vi "Process_One_Second.vi"(6 "Queues":T12, 7 "One Seconds in":T10[](array[typedef]) {"Ch1 High" format="%0.0f"}, 8 "Status/Errors in":refnum<vi>, 9 "Process data parameters in":T1={"Stop loop"={"Settings changed?"=FALSE, "Stop?"=refnum}, "Button refs"={"Stop program"=refnum, "Save settings"=refnum, "DAQ mode"=refnum, "Reset settings"=refnum, "Apply settings"=refnum, "Reset MAS"=refnum, "Reset SLV"=refnum, "Local DBase?"=refnum, "Last value DBase"=FALSE, "Database"=refnum, "Calibration"=refnum, "Save settings 2"=refnum}, "Process messages"={"Process message mode"=enum."Error", "Slave data?"=FALSE, "Length get settings message"=0, "Delta time"=0.0, "Data_Filter"={"Filter_Data"=FALSE, "Use_Thresh"=FALSE, "Reduce data?"=FALSE}, "Time_difference_stack"=[], "Starting sec"=0, "Ending sec"=0, "Ending sec 2"=0, "MAS_Page_Thresh"=refnum, "SLV_Page_Thresh"=refnum, "Database"=refnum}, "Settings state"={"MAS locked?"=refnum, "SLV locked?"=refnum}, "Mode"={"Mode"=enum."Dialog", "Expert?"=FALSE, "Dialog?"=FALSE}, "Alignment parameters"=refnum, "Timer parameters"=refnum, "Files"={"Path config file"=path "", "Path def. ini file"=path "", "Path ini file 1"=path "", "Path ini file 2"=path "", "Path RBF file"=path ""}, "Time difference"=refnum, "Alignment"={"GEN_Page_Calibrate"=refnum, "MAS_Page_Gain"=refnum, "MAS_Page_Offset"=refnum, "SLV_Page_Gain"=refnum, "SLV_Page_Offset"=refnum, "MAS_Page_Common"=refnum, "SLV_Page_Common"=refnum}, "Page Statistics"=refnum}, 11 "Device in":refnum<vi>) -> (0 "Status/Errors out":refnum<vi>, 3 "Device out":refnum<vi>, 5 "One Seconds out":T10[](array[typedef]) {"Ch1 High" format="%0.0f"})   [LabVIEW 2010]
uses:
  Controls/Queues.ctl
  Controls/One_Second.ctl
  Controls/GPS_Timestamp.ctl
  Controls/Process_Data_Parameters.ctl
  Controls/Stop_Loop.ctl
  Controls/Button_Refs.ctl
  Controls/Process_Messages.ctl
  Controls/Process_Message_Mode.ctl
  Controls/Settings_State.ctl
  Controls/Mode.ctl
  Controls/Files.ctl
  Controls/Page_Calibration.ctl
  Controls/Device_Elements.ctl
  Controls/Get_Set_Device_Options.ctl
  Controls/Get_Set_Timer_Options.ctl
  Controls/Add_Subtract.ctl
  Controls/Master.ctl
  Controls/Configuration_File_Parameters.ctl
  Controls/Timer_Elements.ctl
  Controls/Configuration_File_Elements.ctl
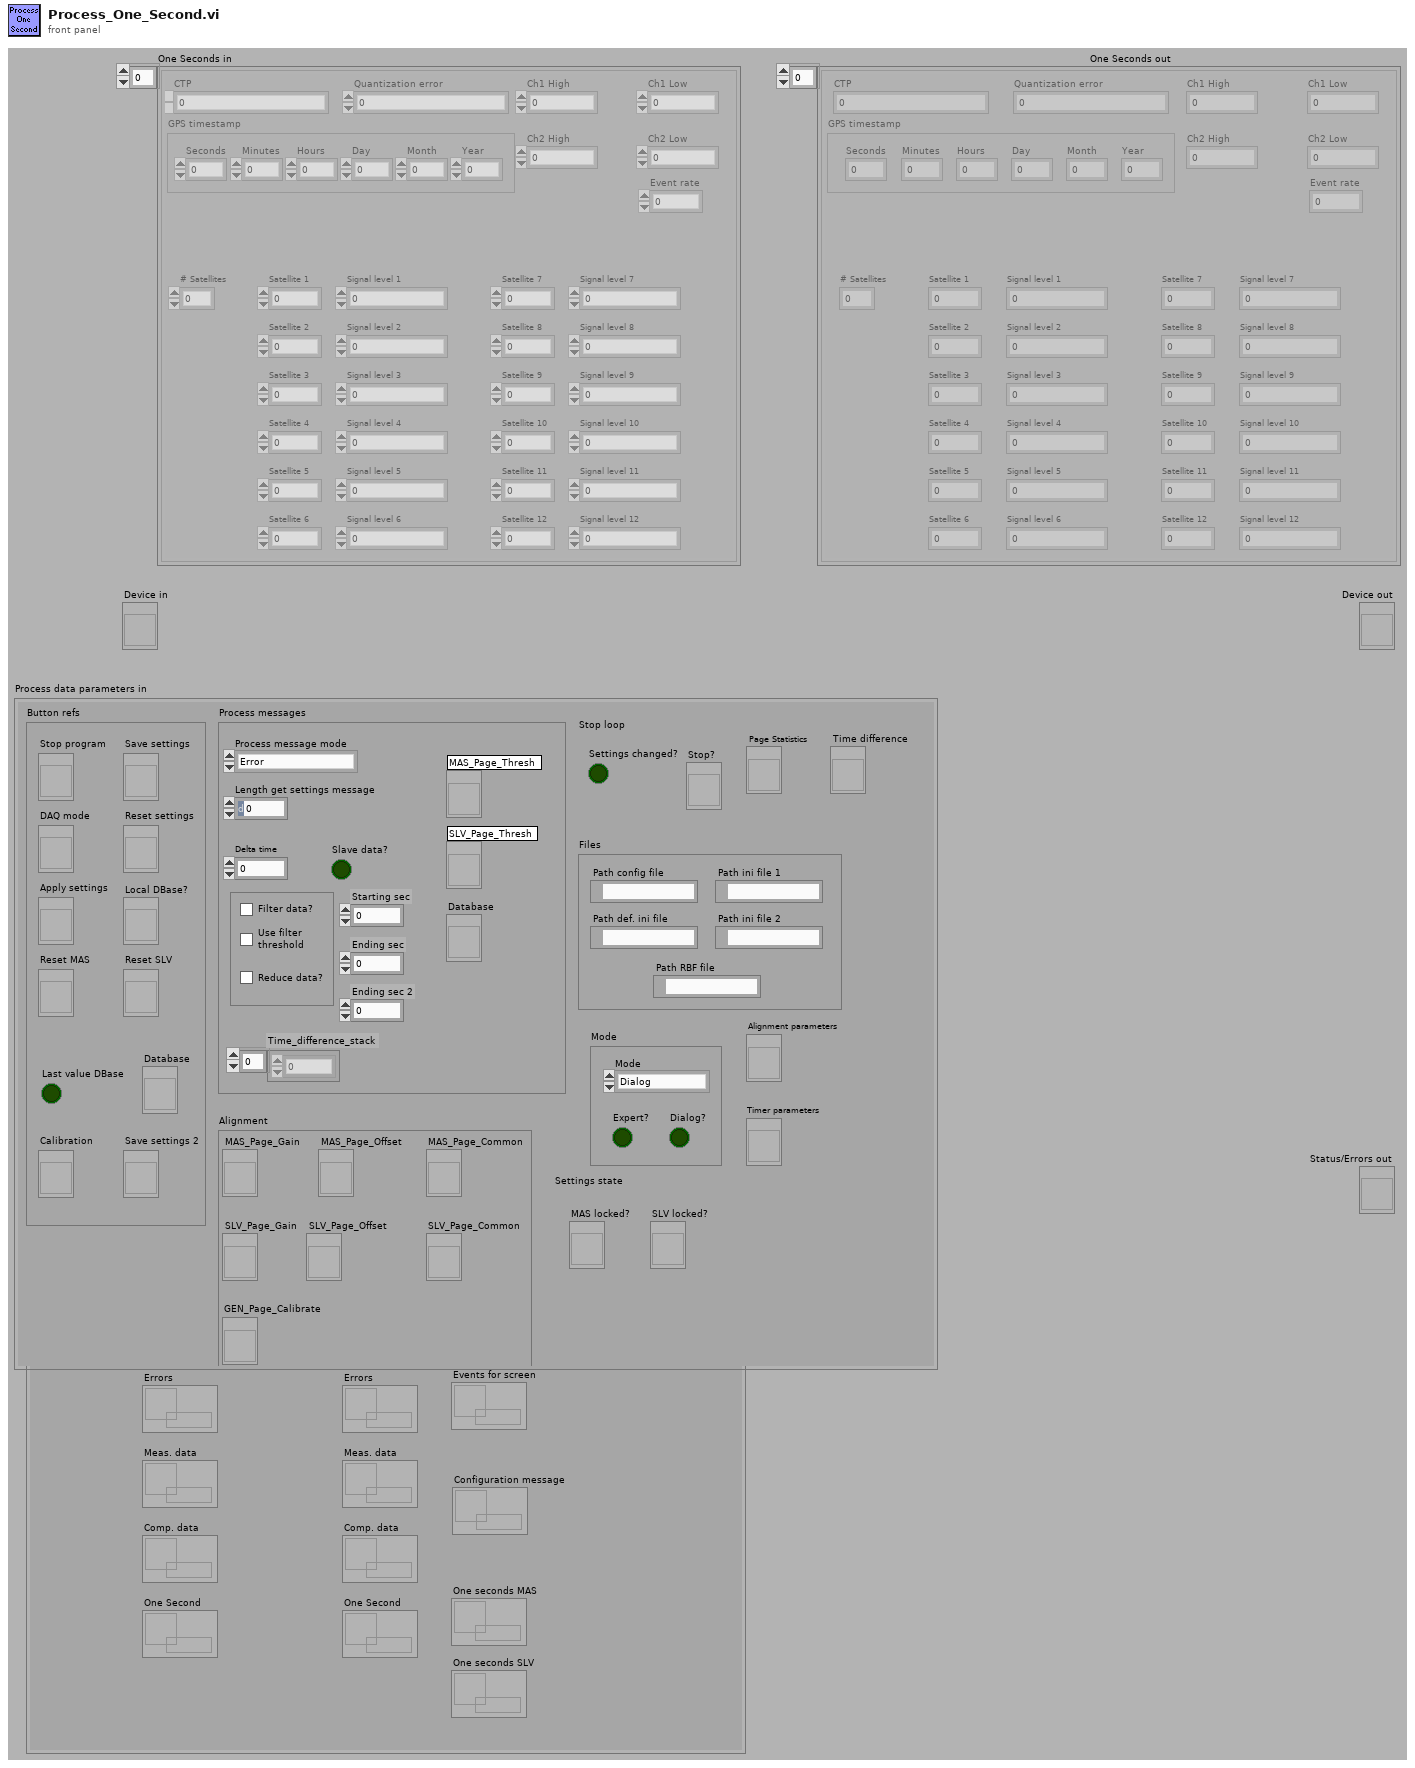
[diagram p1: front panel]
types:
  T1 = typedef "Process_Data_Parameters.ctl" = cluster{"Stop loop":T2, "Button refs":T3, "Process messages":T4, "Settings state":T6, "Mode":T7, "Alignment parameters":refnum<vi>, "Timer parameters":refnum<vi>, "Files":T8, "Time difference":refnum<vi>, "Alignment":T9, "Page Statistics":refnum<vi>}
  T2 = typedef "Stop_Loop.ctl" = cluster{"Settings changed?":bool, "Stop?":refnum<vi>}
  T3 = typedef "Button_Refs.ctl" = cluster{"Stop program":refnum<vi>, "Save settings":refnum<vi>, "DAQ mode":refnum<vi>, "Reset settings":refnum<vi>, "Apply settings":refnum<vi>, "Reset MAS":refnum<vi>, "Reset SLV":refnum<vi>, "Local DBase?":refnum<vi>, "Last value DBase":bool, "Database":refnum<vi>, "Calibration":refnum<vi>, "Save settings 2":refnum<vi>}
  T4 = typedef "Process_Messages.ctl" = cluster{"Process message mode":T5, "Slave data?":bool, "Length get settings message":i32, "Delta time":dbl, "Data_Filter":cluster{"Filter_Data":bool, "Use_Thresh":bool, "Reduce data?":bool}, "Time_difference_stack":u64[], "Starting sec":u64, "Ending sec":u64, "Ending sec 2":u64, "MAS_Page_Thresh":refnum<vi>, "SLV_Page_Thresh":refnum<vi>, "Database":refnum<vi>}
  T5 = typedef "Process_Message_Mode.ctl" = enum16{"Error", "Measurement data", "Comparator data", "One Second"}
  T6 = typedef "Settings_State.ctl" = cluster{"MAS locked?":refnum<vi>, "SLV locked?":refnum<vi>}
  T7 = typedef "Mode.ctl" = cluster{"Mode":enum8{"Stop", "Dialog", "Hisparc II", "Hisparc II DAQ", "Alignment"}, "Expert?":bool, "Dialog?":bool}
  T8 = typedef "Files.ctl" = cluster{"Path config file":path, "Path def. ini file":path, "Path ini file 1":path, "Path ini file 2":path, "Path RBF file":path}
  T9 = typedef "Page_Calibration.ctl" = cluster{"GEN_Page_Calibrate":refnum<vi>, "MAS_Page_Gain":refnum<vi>, "MAS_Page_Offset":refnum<vi>, "SLV_Page_Gain":refnum<vi>, "SLV_Page_Offset":refnum<vi>, "MAS_Page_Common":refnum<vi>, "SLV_Page_Common":refnum<vi>}
  T10 = typedef "One_Second.ctl" = cluster{"GPS timestamp":T11, "CTP":u32, "Quantization error":u32, "Ch1 High":u16, "Ch1 Low":u16, "Ch2 High":u16, "Ch2 Low":u16, "Event rate":u16, "# Satellites":u8, "Satellite 1":u8, "Satellite 2":u8, "Satellite 3":u8, "Satellite 4":u8, "Satellite 5":u8, "Satellite 6":u8, "Signal level 1":sgl, "Signal level 2":sgl, "Signal level 3":sgl, "Signal level 4":sgl, "Signal level 5":sgl, "Signal level 6":sgl, "Satellite 7":u8, "Satellite 8":u8, "Satellite 9":u8, "Satellite 10":u8, "Satellite 11":u8, "Satellite 12":u8, "Signal level 7":sgl, "Signal level 8":sgl, "Signal level 9":sgl, "Signal level 10":sgl, "Signal level 11":sgl, "Signal level 12":sgl}
  T11 = typedef "GPS_Timestamp.ctl" = cluster{"Seconds":u8, "Minutes":u8, "Hours":u8, "Day":u8, "Month":u8, "Year":u16}
  T12 = typedef "Queues.ctl" = cluster{"MAS":cluster{"Bytes":refnum<queue>, "Settings":refnum<queue>, "Errors":refnum<queue>, "Meas. data":refnum<queue>, "One Second":refnum<queue>, "Comp. data":refnum<queue>}, "SLV":cluster{"Bytes":refnum<queue>, "Settings":refnum<queue>, "Errors":refnum<queue>, "Meas. data":refnum<queue>, "One Second":refnum<queue>, "Comp. data":refnum<queue>}, "Events to store":refnum<queue>, "Events for screen":refnum<queue>, "One seconds MAS":refnum<queue>, "One seconds SLV":refnum<queue>, "Configuration message":refnum<queue>, "Comparator to store":refnum<queue>}
  T13 = typedef "Get_Set_Device_Options.ctl" = enum16{"Get", "Get cluster", "Set"}
  T14 = typedef "Device_Elements.ctl" = enum16{"Default", "Master?", "Connected?", "Status", "Disconnect?", "Handle", "Version number"}
  T15 = typedef "Master.ctl" = enum16{"Master", "Slave", "General"}
  T16 = typedef "Get_Set_Timer_Options.ctl" = enum16{"Get", "Get cluster", "Set", "Set to current time"}
  T17 = typedef "Timer_Parameters.ctl" = cluster{"current time (ms)":u32, "time (ms) screen updated":u32, "time (ms) controls locked":u32, "time (ms) last device check":u32, "time (ms) last data MAS":u32, "time (ms) last data SLV":u32, "time (ms) bad status MAS":u32, "time (ms) bad status SLV":u32, "time (ms) clock error updated":u32, "time delay screen update (ms)":u32, "time delay controls (ms)":u32, "time delay device check (ms)":u32, "time until MAS status bad (ms)":u32, "time until SLV status bad (ms)":u32, "time until MAS connection bad (ms)":u32, "time until SLV connection bad (ms)":u32, "time delay clock error update (ms)":u32}
  T18 = cluster{"[0]":u8, "[1]":u8, "[2]":u8, "[3]":u8, "[4]":u8, "[5]":u8, "[6]":u8}
  T19 = cluster{"[0]":u8, "[1]":u8, "[2]":u8, "[3]":u8, "[4]":u8, "[5]":u8, "[6]":u8, "[7]":u8}
  T20 = cluster{"second":i32, "minute":i32, "hour":i32, "day of month":i32, "month":i32, "year":i32, "day of week":i32, "day of year":i32, "is DST":i32}
  T21 = typedef "Add_Subtract.ctl" = enum16{"Add", "Subtract"}
  T22 = typedef "Configuration_File_Parameters.ctl" = cluster{"Mode":T7, "Hardware":enum8{"None", "HiSPARC I", "HiSPARC II", "HiSPARC III"}, "Time difference":string}
  T23 = typedef "Timer_Elements.ctl" = enum16{"Default", "Current time", "Time screen updated", "Time controls locked", "Time last device check", "Time last data MAS", "Time last data SLV", "Time bad status MAS", "Time bad status SLV", "Time clock error updated", "Time delay screen update", "Time delay controls", "Time delay device check", "Time until MAS status bad", "Time until SLV status bad", "Time until MAS connection bad", "Time until SLV connection bad", "Time delay clock error update"}
  T24 = typedef "Configuration_File_Elements.ctl" = enum16{"None", "All", "Mode", "Hardware", "Time difference"}
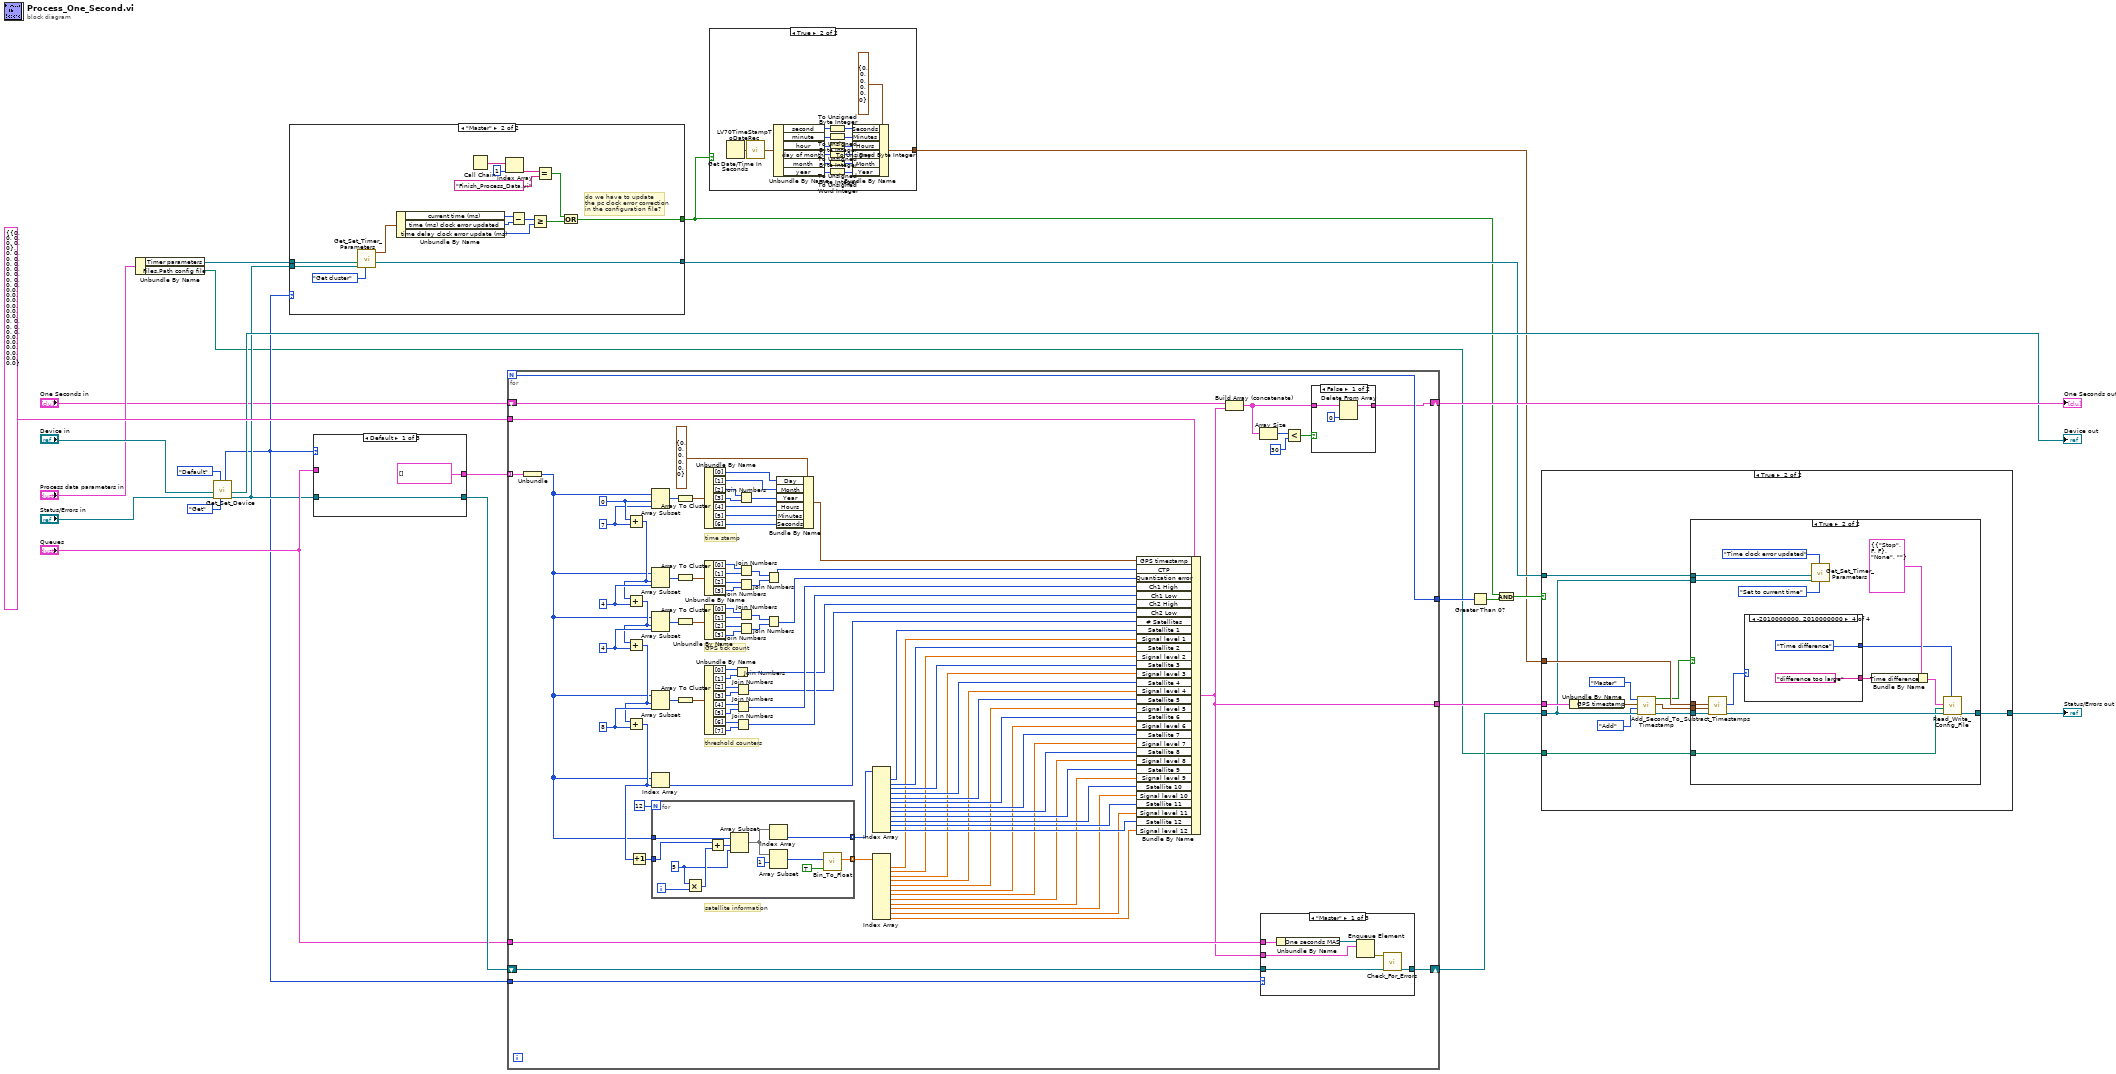
[diagram p0: block diagram]
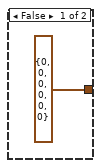
[diagram p2: hidden frame]
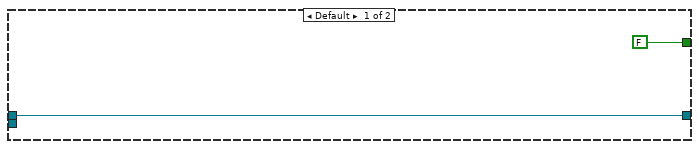
[diagram p3: hidden frame]
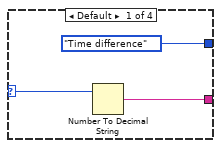
[diagram p6: hidden frame]
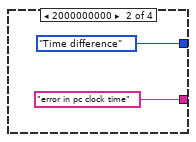
[diagram p7: hidden frame]
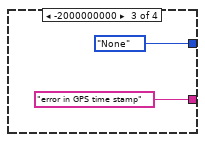
[diagram p8: hidden frame]
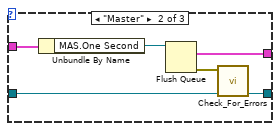
[diagram p9: hidden frame]
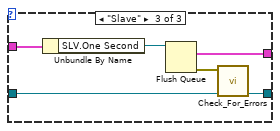
[diagram p10: hidden frame]
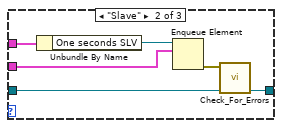
[diagram p12: hidden frame]
diagram:
  n1 = Unbundle By Name("Process data parameters in") -> ("Timer parameters"=w5:refnum<vi>, "Files.Path config file"=w1:path)
  n2 = call "Get_Set_Device.vi"("Get/Set"=Get_Set_Device_Options."Get", "Element"=Device_Elements."Default", "Status/Errors in"="Status/Errors in", "Device in"="Device in") -> ("Status/Errors out"=w8:refnum<vi>, "Device out"=→"Device out":refnum<vi>, "Master?"=w7:T15)  [unwired: 1 in, 4 out]
  n3 = case shown="\"Master\"" w7 {
    tunnel: w5 -> [w26 w33]
    tunnel: [w26 w38] -> w11
    tunnel: [FALSE w35] -> w4
    tunnel: w8 -> [_ w34]
    frame Default {
    }
    frame "Master" {
      # "do we have to update\nthe pc clock error correction\nin the configuration file?"
      n4 = call "Get_Set_Timer_Parameters.vi"("Get/Set"=Get_Set_Timer_Options."Get cluster", "Status/Errors in"=w34, "Timer parameters in"=w33) -> ("Timer parameters out"=w38:refnum<vi>, "Timer cluster"=w37:T17)  [unwired: 2 in, 5 out]
      n5 = Unbundle By Name(w37) -> ("current time (ms)"=w29:u32, "time (ms) clock error updated"=w30:u32, "time delay clock error update (ms)"=w31:u32)
      n6 = Call Chain() -> (call chain=w43:string[])
      n7 = Index Array(array=w43, index=1) -> (element=w41:string)
      n8 = Subtract(x=w29, y=w30) -> (x-y=w32:u32)
      n9 = Greater Or Equal?(x=w32, y=w31) -> (x >= y?=w28:bool)
      n10 = Equal?(x=w41, y="Finish_Process_Data.vi") -> (x = y?=w36:bool)
      n11 = Or(x=w36, y=w28) -> (x .or. y?=w35:bool)
    }
  }
  n12 = case shown="Default" w7 {
    tunnel: "Queues" -> [_ w51 w57]
    tunnel: [cluster{u8[]}[] [] ("remaining elements") w50 w56] -> w22
    tunnel: w8 -> [w44 w47 w53]
    tunnel: [w44 w46 w52] -> w20
    frame Default {
    }
    frame "Master" {
      n13 = Unbundle By Name(w51) -> ("MAS.One Second"=w49:refnum<queue>)
      n14 = Flush Queue(queue=w49) -> (remaining elements=w50:cluster{u8[]}[], error out=w48:errorcluster)  [unwired: 1 in, 1 out]
      n15 = call "Check_For_Errors.vi"("Status/Errors in"=w47, "error in"=w48) -> ("Status/Errors out"=w46:refnum<vi>)  [unwired: 9 out]
    }
    frame "Slave" {
      n16 = Unbundle By Name(w57) -> ("SLV.One Second"=w55:refnum<queue>)
      n17 = Flush Queue(queue=w55) -> (remaining elements=w56:cluster{u8[]}[], error out=w54:errorcluster)  [unwired: 1 in, 1 out]
      n18 = call "Check_For_Errors.vi"("Status/Errors in"=w53, "error in"=w54) -> ("Status/Errors out"=w52:refnum<vi>)  [unwired: 9 out]
    }
  }
  n19 = for {
    N -> [w72]
    tunnel: w22 -> [w111] mode=indexing
    shift-right: [w66] -> w23
    shift-left: "One Seconds in" -> [w68]
    tunnel: T10 {"GPS timestamp"={"Seconds"=0, "Minutes"=0, "Hours"=0, "Day"=0, "Month"=0, "Year"=0}, "CTP"=0, "Quantization error"=0, "Ch1 High"=0, "Ch1 Low"=0, "Ch2 High"=0, "Ch2 Low"=0, "Event rate"=0, "# Satellites"=0, "Satellite 1"=0, "Satellite 2"=0, "Satellite 3"=0, "Satellite 4"=0, "Satellite 5"=0, "Satellite 6"=0, "Signal level 1"=0.0, "Signal level 2"=0.0, "Signal level 3"=0.0, "Signal level 4"=0.0, "Signal level 5"=0.0, "Signal level 6"=0.0, "Satellite 7"=0, "Satellite 8"=0, "Satellite 9"=0, "Satellite 10"=0, "Satellite 11"=0, "Satellite 12"=0, "Signal level 7"=0.0, "Signal level 8"=0.0, "Signal level 9"=0.0, "Signal level 10"=0.0, "Signal level 11"=0.0, "Signal level 12"=0.0} ("GPS Tick Count Message") -> [w110]
    tunnel: w7 -> [w75]
    tunnel: "Queues" -> [w74]
    tunnel: [w69] -> w16
    shift-right: [w73] -> w13
    shift-left: w20 -> [w76]
    tunnel: [w72] -> w10
    w109 = 8 ("y")
    w115 = 4 ("y")
    w116 = 4 ("y")
    w117 = 7 ("y")
    w118 = 0
    # "satellite information"
    # "time stamp"
    # "GPS tick count"
    # "threshold counters"
    n20 = Unbundle(w111) -> (w103:u8[])
    n21 = Add(x=w118, y=w117) -> (x+y=w114:i32)
    n22 = Add(x=w114, y=w116) -> (x+y=w113:i32)
    n23 = Add(x=w113, y=w115) -> (x+y=w108:i32)
    n24 = Add(x=w108, y=w109) -> (x+y=w107:i32)
    n25 = Increment(x=w107) -> (x+1=w106:i32)
    n26 = Array Subset(array=w103, index=w118, length=w117) -> (w154:u8[])
    n27 = Array Subset(array=w103, index=w114, length=w116) -> (w129:u8[])
    n28 = Array Subset(array=w103, index=w113, length=w115) -> (w130:u8[])
    n29 = Array Subset(array=w103, index=w108, length=w109) -> (w128:u8[])
    n30 = Index Array(array=w103, index=w107) -> (element=w105:u8)
    n31 = for {
      N: 12 -> [_]
      tunnel: w106 -> [w176]
      tunnel: w103 -> [w179]
      tunnel: [w174] -> w102 mode=indexing
      tunnel: [w173] -> w89 mode=indexing
      i -> [w178]
      w172 = 5 ("x")
      n32 = Multiply(x=w172, y=w178) -> (x*y=w175:i32)
      n33 = Add(x=w176, y=w175) -> (x+y=w177:i32)
      n34 = Array Subset(array=w179, index=w177, length=w172) -> (w183:u8[])
      n35 = Index Array(array=w183) -> (element=w174:u8)  [unwired: 1 in]
      n36 = Array Subset(array=w183, index=1) -> (w181:u8[])  [unwired: 1 in]
      n37 = call "Bin_To_Float.vi"("32 Bit?"=TRUE, "Binary float"=w181) -> ("Single-Precision Float"=w173:sgl)  [unwired: 9 out]
    }
    n38 = Array To Cluster(array=w154) -> (cluster=w138:T18)
    n39 = Array To Cluster(array=w129) -> (cluster=w131:cluster{"[0]":u8, "[1]":u8, "[2]":u8, "[3]":u8})
    n40 = Array To Cluster(array=w130) -> (cluster=w143:cluster{"[0]":u8, "[1]":u8, "[2]":u8, "[3]":u8})
    n41 = Array To Cluster(array=w128) -> (cluster=w123:T19)
    n42 = Unbundle By Name(w138) -> ("[0]"=w150:u8, "[1]"=w149:u8, "[2]"=w152:u8, "[3]"=w151:u8, "[4]"=w147:u8, "[5]"=w146:u8, "[6]"=w112:u8)
    n43 = Unbundle By Name(w131) -> ("[0]"=w134:u8, "[1]"=w136:u8, "[2]"=w135:u8, "[3]"=w137:u8)
    n44 = Unbundle By Name(w143) -> ("[0]"=w142:u8, "[1]"=w140:u8, "[2]"=w141:u8, "[3]"=w139:u8)
    n45 = Unbundle By Name(w123) -> ("[0]"=w127:u8, "[1]"=w125:u8, "[2]"=w126:u8, "[3]"=w124:u8, "[4]"=w122:u8, "[5]"=w121:u8, "[6]"=w120:u8, "[7]"=w119:u8)
    n46 = Join Numbers(hi=w127, lo=w125) -> ((hi.lo)=w59:u16)
    n47 = Join Numbers(hi=w126, lo=w124) -> ((hi.lo)=w58:u16)
    n48 = Join Numbers(hi=w122, lo=w121) -> ((hi.lo)=w61:u16)
    n49 = Join Numbers(hi=w120, lo=w119) -> ((hi.lo)=w60:u16)
    n50 = Join Numbers(hi=w152, lo=w151) -> ((hi.lo)=w148:u16)
    n51 = Join Numbers(hi=w134, lo=w136) -> ((hi.lo)=w132:u16)
    n52 = Join Numbers(hi=w135, lo=w137) -> ((hi.lo)=w133:u16)
    n53 = Join Numbers(hi=w142, lo=w140) -> ((hi.lo)=w145:u16)
    n54 = Join Numbers(hi=w141, lo=w139) -> ((hi.lo)=w144:u16)
    n55 = Join Numbers(hi=w132, lo=w133) -> ((hi.lo)=w63:u32)
    n56 = Join Numbers(hi=w145, lo=w144) -> ((hi.lo)=w62:u32)
    n57 = Bundle By Name(cluster=T11 {"Seconds"=0, "Minutes"=0, "Hours"=0, "Day"=0, "Month"=0, "Year"=0} ("GPS timestamp in"), "Day"=w150, "Month"=w149, "Year"=w148, "Hours"=w147, "Minutes"=w146, "Seconds"=w112) -> (w64:T11)
    n58 = Index Array(array=w102) -> (element #1=w90:u8, element #2=w91:u8, element #3=w92:u8, element #4=w93:u8, element #5=w94:u8, element #6=w95:u8, element #7=w96:u8, element #8=w97:u8, element #9=w98:u8, element #10=w99:u8, element #11=w100:u8, element #12=w101:u8)  [unwired: 12 in]
    n59 = Index Array(array=w89) -> (element #1=w77:sgl, element #2=w78:sgl, element #3=w79:sgl, element #4=w80:sgl, element #5=w81:sgl, element #6=w82:sgl, element #7=w83:sgl, element #8=w84:sgl, element #9=w85:sgl, element #10=w86:sgl, element #11=w87:sgl, element #12=w88:sgl)  [unwired: 12 in]
    n60 = Bundle By Name(cluster=w110, "GPS timestamp"=w64, "CTP"=w63, "Quantization error"=w62, "Ch1 High"=w61, "Ch1 Low"=w60, "Ch2 High"=w59, "Ch2 Low"=w58, "# Satellites"=w105, "Satellite 1"=w90, "Signal level 1"=w77, "Satellite 2"=w91, "Signal level 2"=w78, "Satellite 3"=w92, "Signal level 3"=w79, "Satellite 4"=w93, "Signal level 4"=w80, "Satellite 5"=w94, "Signal level 5"=w81, "Satellite 6"=w95, "Signal level 6"=w82, "Satellite 7"=w96, "Signal level 7"=w83, "Satellite 8"=w97, "Signal level 8"=w84, "Satellite 9"=w98, "Signal level 9"=w85, "Satellite 10"=w99, "Signal level 10"=w86, "Satellite 11"=w100, "Signal level 11"=w87, "Satellite 12"=w101, "Signal level 12"=w88) -> (w69:T10)
    n61 = Build Array (concatenate)(w68, w69) -> (w65:T10[])
    n62 = Array Size(array=w65) -> (size(s)=w71:i32)
    n63 = case shown="\"Master\"" w75 {
      tunnel: w76 -> [w159 w165 w171]
      tunnel: [w164 w170 w171] -> w73
      tunnel: w74 -> [w163 w169 _]
      tunnel: w69 -> [w160 w166 _]
      frame "Master" {
        n64 = Unbundle By Name(w163) -> ("One seconds MAS"=w162:refnum<queue>)
        n65 = Enqueue Element(queue=w162, element=w160) -> (error out=w161:errorcluster)  [unwired: 1 in, 3 out]
        n66 = call "Check_For_Errors.vi"("Status/Errors in"=w159, "error in"=w161) -> ("Status/Errors out"=w164:refnum<vi>)  [unwired: 9 out]
      }
      frame "Slave" {
        n67 = Unbundle By Name(w169) -> ("One seconds SLV"=w168:refnum<queue>)
        n68 = Enqueue Element(queue=w168, element=w166) -> (error out=w167:errorcluster)  [unwired: 1 in, 3 out]
        n69 = call "Check_For_Errors.vi"("Status/Errors in"=w165, "error in"=w167) -> ("Status/Errors out"=w170:refnum<vi>)  [unwired: 9 out]
      }
      frame Default {
      }
    }
    n70 = Less?(x=w71, y=30 ("x")) -> (x < y?=w67:bool)
    n71 = case shown="False" w67 {
      tunnel: [w156 w158] -> w66
      tunnel: w65 -> [w157 w158]
      frame False {
        n72 = Delete From Array(array=w157, index=0) -> (array with subset deleted=w156:T10[])  [unwired: 1 in, 1 out]
      }
      frame True {
      }
    }
  }
  "One Seconds out" <- w23
  n73 = case shown="True" w4 {
    tunnel: [T11 {"Seconds"=0, "Minutes"=0, "Hours"=0, "Day"=0, "Month"=0, "Year"=0} ("GPS timestamp") w186] -> w3
    frame False {
    }
    frame True {
      n74 = Get Date/Time In Seconds() -> (seconds since 1Jan1904=w185:timestamp)
      n75 = call <vilib>:"LV70TimeStampToDateRec.vi"("time stamp"=w185) -> ("date time rec"=w200:T20)
      n76 = Unbundle By Name(w200) -> ("second"=w198:i32, "minute"=w197:i32, "hour"=w196:i32, "day of month"=w195:i32, "month"=w194:i32, "year"=w193:i32)
      n77 = To Unsigned Byte Integer(number=w198) -> (unsigned 8bit integer=w187:u8)
      n78 = To Unsigned Byte Integer(number=w197) -> (unsigned 8bit integer=w188:u8)
      n79 = To Unsigned Byte Integer(number=w196) -> (unsigned 8bit integer=w189:u8)
      n80 = To Unsigned Byte Integer(number=w195) -> (unsigned 8bit integer=w190:u8)
      n81 = To Unsigned Byte Integer(number=w194) -> (unsigned 8bit integer=w191:u8)
      n82 = To Unsigned Word Integer(number=w193) -> (unsigned 16bit integer=w192:u16)
      n83 = Bundle By Name(cluster=T11 {"Seconds"=0, "Minutes"=0, "Hours"=0, "Day"=0, "Month"=0, "Year"=0} ("GPS timestamp"), "Seconds"=w187, "Minutes"=w188, "Hours"=w189, "Day"=w190, "Month"=w191, "Year"=w192) -> (w186:T11)
    }
  }
  n84 = Greater Than 0?(x=w10) -> (x > 0?=w9:bool)
  n85 = And(x=w4, y=w9) -> (x .and. y?=w15:bool)
  n86 = case shown="True" w15 {
    tunnel: w16 -> [_ w211]
    tunnel: w13 -> [w201 w209]
    tunnel: [w201 w213] -> w14
    tunnel: w11 -> [_ w212]
    tunnel: w3 -> [_ w210]
    tunnel: w1 -> [_ w202]
    frame False {
    }
    frame True {
      n87 = Unbundle By Name(w211) -> ("GPS timestamp"=w207:T11)
      n88 = call "Add_Second_To_Timestamp.vi"("Status/Errors in"=w209, "Add/Subtract"=Add_Subtract."Add", "Time stamp"=w207, "Master?"=Master."Master") -> ("Status/Errors out"=w208:refnum<vi>, "Time stamp out"=w205:T11, "Timestamp OK?"=w203:bool)  [unwired: 5 out]
      n89 = case shown="True" w203 {
        tunnel: [w214 w229] -> w213
        tunnel: w212 -> [_ w227]
        tunnel: w210 -> [_ w225]
        tunnel: w209 -> [_ w218]
        tunnel: w208 -> [w214 w217]
        tunnel: w205 -> [_ w216]
        tunnel: w202 -> [_ w215]
        frame False {
        }
        frame True {
          n90 = call "Subtract_Timestamps.vi"("Status/Errors in"=w217, "Time stamp 2"=w216, "Time stamp 1"=w225) -> ("Status/Errors out"=w221:refnum<vi>, "Difference"=w222:i32)  [unwired: 7 out]
          n91 = case shown="-2010000000, 2010000000" w222 {
            selector: w222 -> [w232 _ _ _]
            tunnel: [w231 "error in pc clock time" "error in GPS time stamp" "difference too large"] -> w220
            tunnel: [Configuration_File_Elements."Time difference" ("Element (None)") Configuration_File_Elements."Time difference" ("Element (None)") Configuration_File_Elements."None" ("Element (None)") Configuration_File_Elements."Time difference" ("Element (None)")] -> w219
            frame Default {
              n92 = Number To Decimal String(number=w232) -> (decimal integer string=w231:string)  [unwired: 1 out]
            }
            frame 2000000000 {
            }
            frame -2000000000 {
            }
            frame -2010000000, 2010000000 {
            }
          }
          n93 = call "Get_Set_Timer_Parameters.vi"("Get/Set"=Get_Set_Timer_Options."Set to current time", "Element"=Timer_Elements."Time clock error updated", "Status/Errors in"=w218, "Timer parameters in"=w227) -> ()  [unwired: 1 in, 7 out]
          n94 = Bundle By Name(cluster=T22 {"Mode"={"Mode"=enum."Stop", "Expert?"=FALSE, "Dialog?"=FALSE}, "Hardware"=enum."None", "Time difference"=""} ("Parameters in"), "Time difference"=w220) -> (w223:T22)
          n95 = call "Read_Write_Config_File.vi"("Element (None)"=w219, "Status/Errors in"=w221, "Path config file in"=w215, "Parameters in"=w223) -> ("Status/Errors out"=w229:refnum<vi>)  [unwired: 7 out]
        }
      }
    }
  }
  "Status/Errors out" <- w14
